vi "氨氮固定站质控流程.vi"(6 "队列输入NH3":refnum<queue>, 9 "氨氮":bool, 10 "氨氮量程切换":enum32{"H", "L", "AUTO"}(ring)=enum."AUTO") -> (3 "布尔":bool)   [LabVIEW 2016, in "质控单元.lvlib"]
panel:
  out "氨氮中断报警":bool
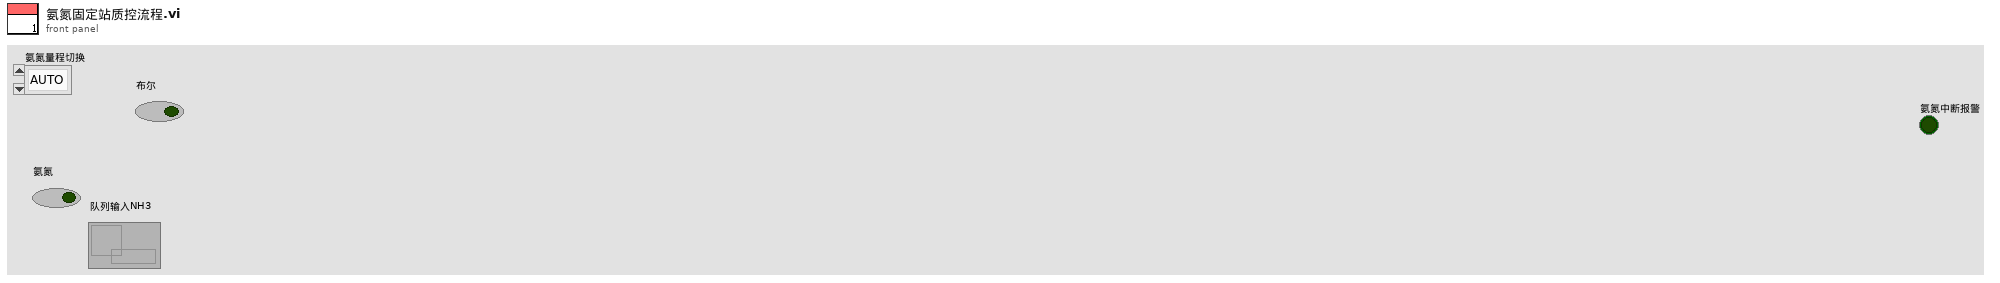
[diagram p1: front panel]
types:
  T1 = enum16{"待机", "启动氨氮水样", "氨氮测量中", "启动氨氮加标", "启动氨氮加标回收", "氨氮加标回收测量中", "启动总氮水样", "总氮测量中", "启动总氮加标", "启动总氮加标回收", "总氮加标回收测量中", "启动总磷水样", "总磷水样测量中", "启动总磷加标", "启动总磷加标回收", "总磷加标回收测量中", "结束"}
  T2 = cluster{"站号":u16, "量程切换":enum32{"H", "L", "AUTO"}, "控制命令":enum16{"启动测量", "标样核查", "零点核查", "跨度核查", "空白测试", "平行样测试", "加标回收", "空白校准", "标样校准", "初始化（清洗）", "停止测试", "仪器重启", "校时", "模式设置", "测量间隔设置"}, "模式设置":enum16{"待机", "连续模式", "周期模式", "定点模式", "受控模式", "手动模式"}, "测量间隔":u16}
  T3 = cluster{"时间标识":timestamp, "设备":string, "日志信息":string}
  T4 = cluster{"系统时间":timestamp, "工作状态":enum16{"空闲", "水样测试", "标样核查", "零点核查", "跨度核查", "空白测试", "平行样测试", "加标回收", "空白校准", "标样校准", "初始化（清洗）"}, "测量模式":enum16{"待机", "连续模式", "周期模式", "定点模式", "受控模式", "手动模式"}, "告警代码":enum16{"无告警", "缺试剂告警", "缺水样告警", "缺蒸馏水告警", "缺标液告警", "仪表漏液告警", "标定异常告警", "超量程告警", "加热异常", "低试剂预警", "超上限告警", "超下限告警", "仪表内部其他异常", "滴定异常告警", "电极异常告警", "量程切换告警", "参数设置告警", "PH电极电位异常", "电导率电极异常", "浊度光度异常", "溶解氧电极异常", "溶解氧光强异常", "温度异常告警", "PH异常告警", "溶解氧异常告警", "电导率异常告警", "浊度异常告警", "叶绿素异常告警", "藻密度异常告警", "蓝绿藻异常告警", "ORP异常告警", "氨氮异常告警", "清洁刷异常告警", "SD卡异常告警", "蓝牙异常告警", "Wifi异常告警", "流程异常告警"}, "故障代码":enum16{"无故障", "电机故障", "温度故障", "通讯故障", "滴定故障"}, "日志代码":u16, "软件版本":u16, "F0":sgl, "F1":sgl, "F2":sgl, "F3":sgl, "T":sgl, "H":sgl, "id":u16, "flowid":u16, "量程":u16, "总磷控温温度1":sgl, "营养盐控温温度2":sgl, "ADC":sgl}
  T5 = enum16{"空闲", "水样测试", "标样核查", "零点核查", "跨度核查", "空白测试", "平行样测试", "加标回收", "空白校准", "标样校准", "初始化（清洗）"}
  T6 = cluster{"量程":dbl, "检出限":dbl, "加标前水样浓度":dbl, "加标后水样浓度":dbl, "加标水杯定容体积":dbl, "加标母液浓度":dbl, "加标体积":dbl, "加标回收率":dbl}
  T7 = cluster{"因子编码":u32, "单位":u16, "标样参考值":sgl, "水样数据时间":timestamp, "水样实测值":sgl, "水样数据标识":string, "标样数据时间":timestamp, "标样实测值":sgl, "标样数据标识":string, "空白数据时间":timestamp, "空白实测值":sgl, "空白数据标识":string, "零点核查数据时间":timestamp, "零点核查实测值":sgl, "零点核查数据标识":string, "跨度核查数据时间":timestamp, "跨度核查实测值":sgl, "跨度核查数据标识":string, "加标回收数据时间":timestamp, "加标回收实测值":sgl, "加标回收数据标识":string, "平行样数据时间":timestamp, "平行样实测值":sgl, "平行样数据标识":string}
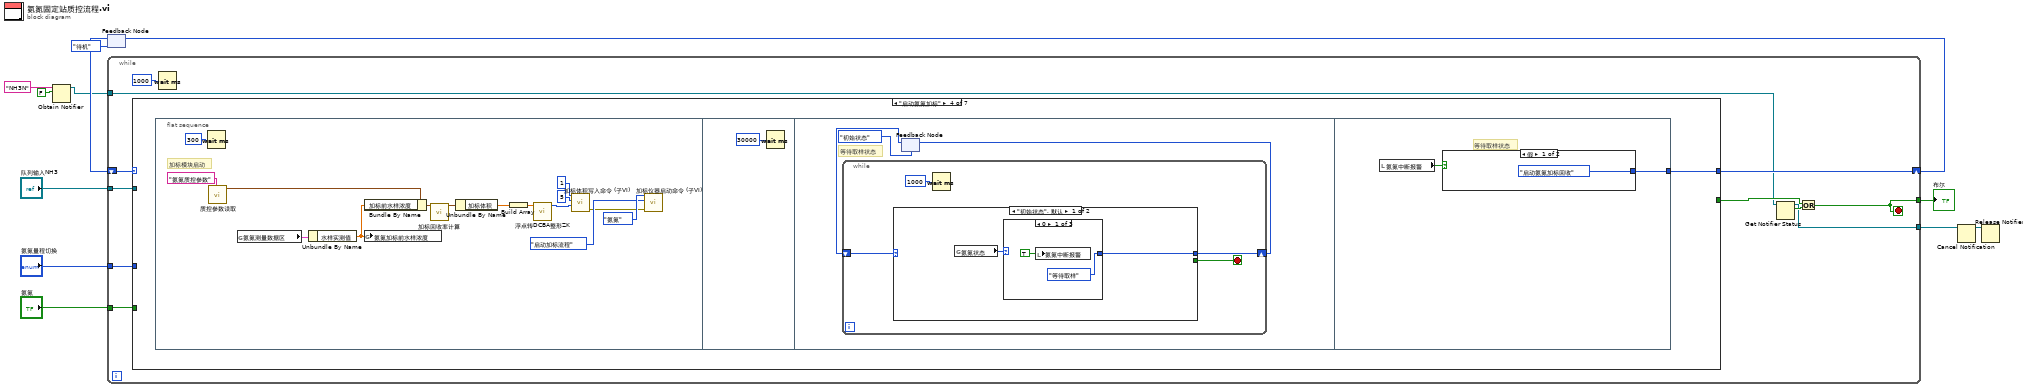
[diagram p0: block diagram]
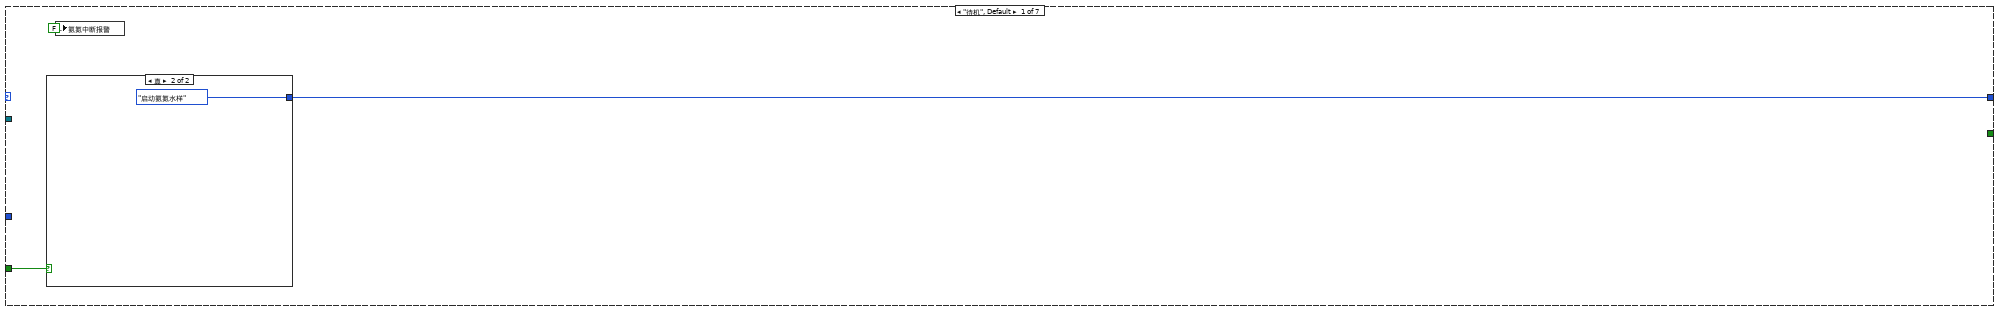
[diagram p2: hidden frame]
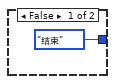
[diagram p3: hidden frame]
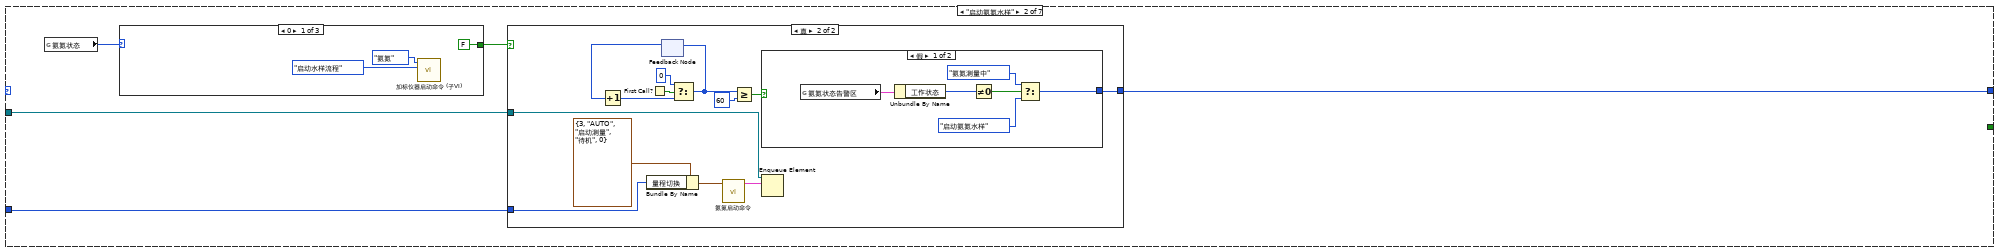
[diagram p4: hidden frame]
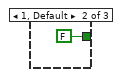
[diagram p5: hidden frame]
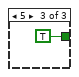
[diagram p6: hidden frame]
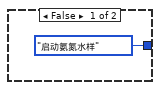
[diagram p7: hidden frame]
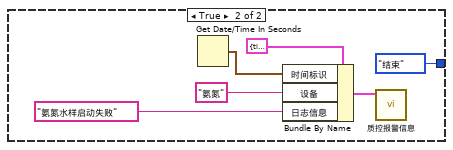
[diagram p8: hidden frame]
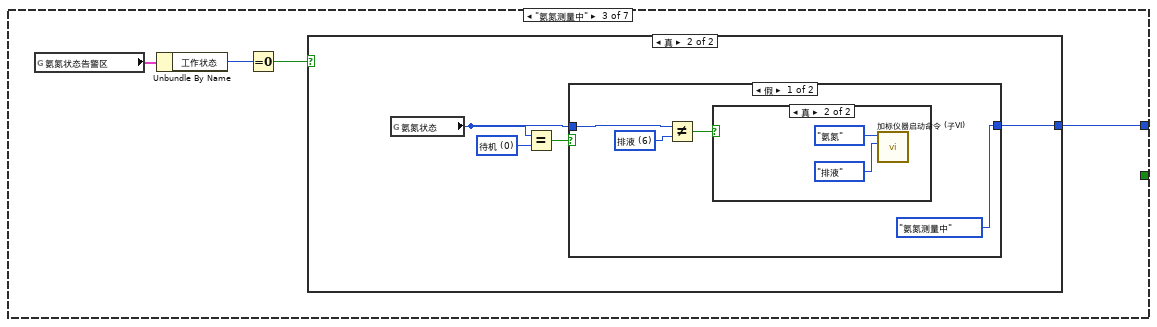
[diagram p9: hidden frame]
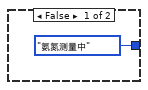
[diagram p10: hidden frame]
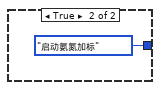
[diagram p12: hidden frame]
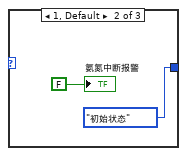
[diagram p13: hidden frame]
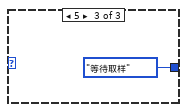
[diagram p14: hidden frame]
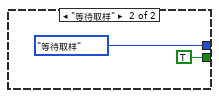
[diagram p15: hidden frame]
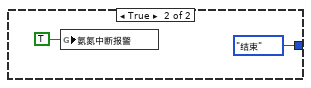
[diagram p16: hidden frame]
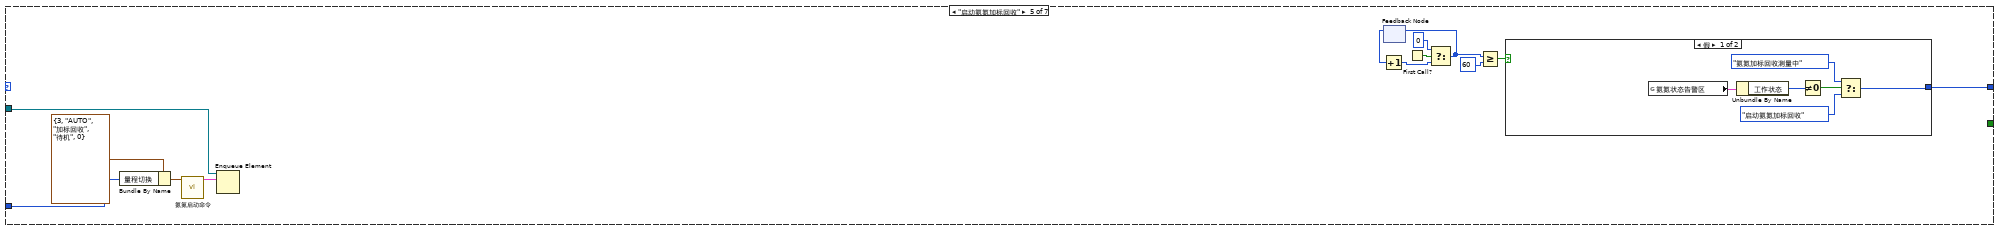
[diagram p17: hidden frame]
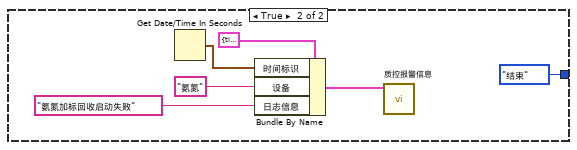
[diagram p18: hidden frame]
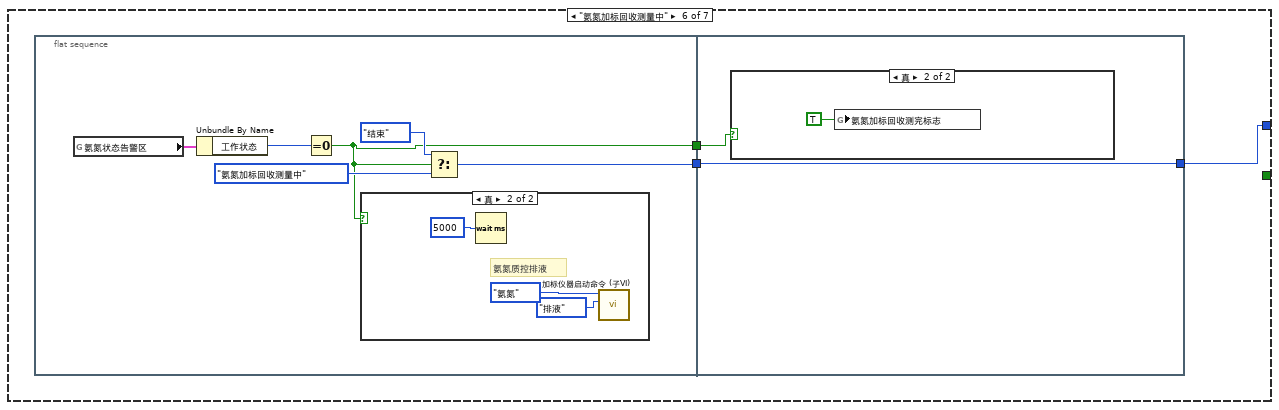
[diagram p19: hidden frame]
diagram:
  n1 = Obtain Notifier(name (unnamed)="NH3N" ("名称（未命名）"), notification data type=FALSE) -> (notifier out=w3:refnum<notifier>)  [unwired: 2 in, 2 out]
  n2 = feedback #1(T1."待机") -> (w6:T1)
  n3 = while {
    tunnel: "队列输入NH3" -> [w21]
    tunnel: "氨氮量程切换" -> [w20]
    tunnel: "氨氮" -> [w23]
    tunnel: [w15] -> w11
    shift-right: [w22] -> w9
    shift-left: w6 -> [w19]
    tunnel: w3 -> [w14]
    tunnel: [w13] -> w1
    stop <- w15 stop-if-true
    n4 = case shown="\"启动氨氮加标\"" w19 {
      tunnel: [w26 w33 w65 w81 w124 w145 T1."结束"] -> w22
      tunnel: [_ _ _ _ _ _ TRUE] -> w16
      tunnel: w23 -> [w25 _ _ _ _ _ _]
      tunnel: w21 -> [_ w32 _ _ w122 _ _]
      tunnel: w20 -> [_ w31 _ _ w119 _ _]
      frame "待机", Default {
        n5 = case shown="真" w25 {
          tunnel: [T1."结束" T1."启动氨氮水样"] -> w26
          frame False {
          }
          frame True {
          }
        }
        n6 = local write "氨氮中断报警"(FALSE ("氨氮中断报警")) -> ()
      }
      frame "启动氨氮水样" {
        n7 = global read "加标回收状态全局变量.vi" "氨氮状态"() -> (w30:u16)
        n8 = case shown="0" w30 {
          tunnel: [FALSE ("s") FALSE ("s") TRUE ("s")] -> w29
          frame 0 {
            n9 = call "加标仪器启动命令 (子VI).vi"("启动命令"=enum16{"启动水样流程", "启动加标流程", "排液", "停止"}."启动水样流程", "仪器"=enum16{"", "氨氮", "总磷", "总氮", "CODMn", "CODCr"}."氨氮") -> ()  [unwired: 9 in, 1 out]
          }
          frame 1, Default {
          }
          frame 5 {
          }
        }
        n10 = case shown="真" w29 {
          tunnel: [T1."启动氨氮水样" w52] -> w33
          tunnel: w32 -> [_ w43]
          tunnel: w31 -> [_ w40]
          frame False {
          }
          frame True {
            n11 = Bundle By Name(cluster=T2 {"站号"=3, "量程切换"=enum."AUTO", "控制命令"=enum."启动测量", "模式设置"=enum."待机", "测量间隔"=0} ("参数"), "量程切换"=w40) -> (w41:T2)
            n12 = First Call?() -> (First Call?: T/F=w50:bool)
            n13 = feedback #2() -> (w49:i32)  [unwired: 1 in]
            n14 = Increment(x=w49) -> (x+1=w48:i32)
            n15 = Select(t=0, s=w50, f=w48) -> (s? t:f=w47:i32)
            n16 = feedback-in #2(w47) -> ()
            n17 = call "氨氮启动命令.vi"("参数"=w41) -> ("启动命令"=w44:cluster{"命令":string, "data":variant})  [unwired: 10 in]
            n18 = Greater Or Equal?(x=w47, y=60) -> (x >= y?=w45:bool)
            n19 = case shown="假" w45 {
              tunnel: [w56 T1."结束"] -> w52
              frame False {
                n20 = global read "与氨氮交互全局.vi" "氨氮状态告警区"() -> (w53:T4)
                n21 = Unbundle By Name(w53) -> ("工作状态"=w58:T5)
                n22 = Not Equal To 0?(x=w58) -> (x != 0?=w57:bool)
                n23 = Select(t=T1."氨氮测量中", s=w57, f=T1."启动氨氮水样") -> (s? t:f=w56:T1)
              }
              frame True {
                n24 = Get Date/Time In Seconds() -> (seconds since 1Jan1904=w64:timestamp)
                n25 = Bundle By Name(cluster=T3 {"时间标识"=timestamp(0 s since 1904-01-01), "设备"="", "日志信息"=""} ("data in"), "时间标识"=w64, "设备"="氨氮", "日志信息"="氨氮水样启动失败") -> (w59:T3)
                n26 = call "质控报警信息.vi"("data in"=w59) -> ()  [unwired: 10 in, 1 out]
              }
            }
            n27 = Enqueue Element(queue=w43, element=w44) -> ()  [unwired: 2 in, 3 out]
          }
        }
      }
      frame "氨氮测量中" {
        n28 = global read "与氨氮交互全局.vi" "氨氮状态告警区"() -> (w67:T4)
        n29 = Unbundle By Name(w67) -> ("工作状态"=w68:T5)
        n30 = Equal To 0?(x=w68) -> (x = 0?=w66:bool)
        n31 = case shown="真" w66 {
          tunnel: [T1."氨氮测量中" w71] -> w65
          frame False {
          }
          frame True {
            w73 = u16 0 items=["待机", "润洗", "进样", "进样完成", "柱塞泵加标", "等待取液", "排液"] ("氨氮状态")
            n32 = global read "加标回收状态全局变量.vi" "氨氮状态"() -> (w70:u16)
            n33 = Equal?(x=w70, y=w73) -> (x = y?=w72:bool)
            n34 = case shown="假" w72 {
              tunnel: [T1."氨氮测量中" T1."启动氨氮加标"] -> w71
              tunnel: w70 -> [w76 _]
              frame False {
                w75 = u16 6 items=["待机", "润洗", "进样", "进样完成", "柱塞泵加标", "等待取液", "排液"] ("氨氮状态")
                n35 = Not Equal?(x=w76, y=w75) -> (x != y?=w74:bool)
                n36 = case shown="真" w74 {
                  frame False {
                  }
                  frame True {
                    n37 = call "加标仪器启动命令 (子VI).vi"("启动命令"=enum16{"启动水样流程", "启动加标流程", "排液", "停止"}."排液", "仪器"=enum16{"", "氨氮", "总磷", "总氮", "CODMn", "CODCr"}."氨氮") -> ()  [unwired: 9 in, 1 out]
                  }
                }
              }
              frame True {
              }
            }
          }
        }
      }
      frame "启动氨氮加标" {
        n38 = flat-sequence {
          tunnel: [w115] -> w81
          frame #0 {
            # "加标模块启动"
            n39 = Wait (ms)(milliseconds to wait=u32 300 ("等待时间（毫秒）")) -> ()  [unwired: 1 out]
            n40 = call "质控参数读取.vi"("section"="氨氮质控参数") -> ("参数"=w95:T6)  [unwired: 9 in, 1 out]
            n41 = global read "与氨氮交互全局.vi" "氨氮测量数据区"() -> (w82:T7)
            n42 = Unbundle By Name(w82) -> ("水样实测值"=w83:sgl)
            n43 = Bundle By Name(cluster=w95, "加标前水样浓度"=w83) -> (w85:T6)
            n44 = global write "水样浓度全局.vi" "氨氮加标前水样浓度"(w83) -> ()
            n45 = call "加标回收率计算.vi"("参数"=w85) -> ("参数 out"=w84:T6)  [unwired: 9 in, 1 out]
            n46 = Unbundle By Name(w84) -> ("加标体积"=w94:dbl)
            n47 = Build Array(w94) -> (w92:dbl[])
            n48 = call "浮点转DCBA整形ZK.vi"("浮点数"=w92) -> ("DCBA整形输出"=w86:u16[])  [unwired: 10 in]
            n49 = call "加标体积写入命令 (子VI).vi"("values"=w86, "starting address"=u16 5, "Slave ID"=u16 1 ("value")) -> ("错误输出"=w89:errorcluster)  [unwired: 8 in]
            n50 = call "加标仪器启动命令 (子VI).vi"("错误输入（无错误）"=w89, "启动命令"=enum16{"启动水样流程", "启动加标流程", "排液", "停止"}."启动加标流程", "仪器"=enum16{"", "氨氮", "总磷", "总氮", "CODMn", "CODCr"}."氨氮") -> ()  [unwired: 8 in, 1 out]
          }
          frame #1 {
            n51 = Wait (ms)(milliseconds to wait=u32 30000 ("等待时间（毫秒）")) -> ()  [unwired: 1 out]
          }
          frame #2 {
            # "等待取样状态"
            n52 = feedback #3(enum16{"初始状态", "等待取样"}."初始状态") -> (w99:enum16{"初始状态", "等待取样"})
            n53 = while {
              shift-right: [w103] -> w98
              shift-left: w99 -> [w104]
              stop <- w102 stop-if-true
              n54 = case shown="\"初始状态\", 默认" w104 {
                tunnel: [w106 enum16{"初始状态", "等待取样"}."等待取样"] -> w103
                tunnel: [_ TRUE] -> w102
                frame "初始状态", Default {
                  n55 = global read "加标回收状态全局变量.vi" "氨氮状态"() -> (w105:u16)
                  n56 = case shown="0" w105 {
                    tunnel: [enum16{"初始状态", "等待取样"}."等待取样" enum16{"初始状态", "等待取样"}."初始状态" enum16{"初始状态", "等待取样"}."等待取样"] -> w106
                    frame 0 {
                      n57 = local write "氨氮中断报警"(TRUE ("氨氮中断报警")) -> ()
                    }
                    frame 1, Default {
                      "氨氮中断报警" <- FALSE ("总氮中断报警")
                    }
                    frame 5 {
                    }
                  }
                }
                frame "等待取样" {
                }
              }
              n58 = Wait (ms)(milliseconds to wait=u32 1000 ("等待时间（毫秒）")) -> ()  [unwired: 1 out]
            }
            n59 = feedback-in #3(w98) -> ()
          }
          frame #3 {
            # "等待取样状态"
            n60 = local read "氨氮中断报警"() -> (w114:bool)
            n61 = case shown="假" w114 {
              tunnel: [T1."启动氨氮加标回收" T1."结束"] -> w115
              frame False {
              }
              frame True {
                n62 = global write "质控中断报警全局.vi" "氨氮中断报警"(TRUE ("氨氮中断报警")) -> ()
              }
            }
          }
        }
      }
      frame "启动氨氮加标回收" {
        n63 = Bundle By Name(cluster=T2 {"站号"=3, "量程切换"=enum."AUTO", "控制命令"=enum."加标回收", "模式设置"=enum."待机", "测量间隔"=0} ("参数"), "量程切换"=w119) -> (w120:T2)
        n64 = call "氨氮启动命令.vi"("参数"=w120) -> ("启动命令"=w123:cluster{"命令":string, "data":variant})  [unwired: 10 in]
        n65 = Enqueue Element(queue=w122, element=w123) -> ()  [unwired: 2 in, 3 out]
        n66 = feedback #4() -> (w129:i32)  [unwired: 1 in]
        n67 = Increment(x=w129) -> (x+1=w128:i32)
        n68 = First Call?() -> (First Call?: T/F=w130:bool)
        n69 = Select(t=0, s=w130, f=w128) -> (s? t:f=w127:i32)
        n70 = feedback-in #4(w127) -> ()
        n71 = Greater Or Equal?(x=w127, y=60) -> (x >= y?=w125:bool)
        n72 = case shown="假" w125 {
          tunnel: [w135 T1."结束"] -> w124
          frame False {
            n73 = global read "与氨氮交互全局.vi" "氨氮状态告警区"() -> (w132:T4)
            n74 = Unbundle By Name(w132) -> ("工作状态"=w137:T5)
            n75 = Not Equal To 0?(x=w137) -> (x != 0?=w136:bool)
            n76 = Select(t=T1."氨氮加标回收测量中", s=w136, f=T1."启动氨氮加标回收") -> (s? t:f=w135:T1)
          }
          frame True {
            n77 = Get Date/Time In Seconds() -> (seconds since 1Jan1904=w143:timestamp)
            n78 = Bundle By Name(cluster=T3 {"时间标识"=timestamp(0 s since 1904-01-01), "设备"="", "日志信息"=""} ("data in"), "时间标识"=w143, "设备"="氨氮", "日志信息"="氨氮加标回收启动失败") -> (w138:T3)
            n79 = call "质控报警信息.vi"("data in"=w138) -> ()  [unwired: 10 in, 1 out]
          }
        }
      }
      frame "氨氮加标回收测量中" {
        n80 = flat-sequence {
          tunnel: [w151] -> w146
          tunnel: [w147] -> w144
          tunnel: [w157] -> w145
          tunnel: w146 -> [w157]
          tunnel: w144 -> [w156]
          frame #0 {
            n81 = global read "与氨氮交互全局.vi" "氨氮状态告警区"() -> (w148:T4)
            n82 = Unbundle By Name(w148) -> ("工作状态"=w152:T5)
            n83 = Equal To 0?(x=w152) -> (x = 0?=w147:bool)
            n84 = case shown="真" w147 {
              frame False {
              }
              frame True {
                # "氨氮质控排液"
                n85 = Wait (ms)(milliseconds to wait=u32 5000 ("等待时间（毫秒）")) -> ()  [unwired: 1 out]
                n86 = call "加标仪器启动命令 (子VI).vi"("启动命令"=enum16{"启动水样流程", "启动加标流程", "排液", "停止"}."排液", "仪器"=enum16{"", "氨氮", "总磷", "总氮", "CODMn", "CODCr"}."氨氮") -> ()  [unwired: 9 in, 1 out]
              }
            }
            n87 = Select(t=T1."结束", s=w147, f=T1."氨氮加标回收测量中") -> (s? t:f=w151:T1)
          }
          frame #1 {
            n88 = case shown="真" w156 {
              frame False {
              }
              frame True {
                n89 = global write "质控测完标志全局 1.vi" "氨氮加标回收测完标志"(TRUE) -> ()
              }
            }
          }
        }
      }
      frame "结束" {
        n90 = Wait (ms)(milliseconds to wait=u32 5000 ("等待时间（毫秒）")) -> ()  [unwired: 1 out]
      }
    }
    n91 = Wait (ms)(milliseconds to wait=u32 1000 ("等待时间（毫秒）")) -> ()  [unwired: 1 out]
    n92 = Get Notifier Status(notifier=w14) -> (notifier out=w13:refnum<notifier>, current notification=w17:bool)  [unwired: 1 in, 3 out]
    n93 = Or(x=w16, y=w17) -> (x .or. y?=w15:bool)
  }
  "布尔" <- w11
  n94 = feedback-in #1(w9) -> ()
  n95 = Cancel Notification(0:w1) -> (8:w2:refnum<notifier>)  [unwired: 1 in, 2 out]
  n96 = Release Notifier(notifier=w2) -> ()  [unwired: 2 in, 3 out]
